vi "Read analyze results.vi"(5 "ChemStation rawdata folder":path=path "C:/Users/Optix/Dropbox (MIT)/Research/Backup/66-225 Optix data/Yiming MO/AC electrolysis/HPLC data backup", 7 "ChemStation folder":path=path "C:/Users/Optix/Dropbox (MIT)/Research/Backup/66-225 Optix data/Yiming MO/AC electrolysis/HPLC data backup", 8 "Index":dbl, 9 "Sample name":string, 10 "Experiment name":string, 11 "Exp. file path":path) -> ()   [LabVIEW 2017]
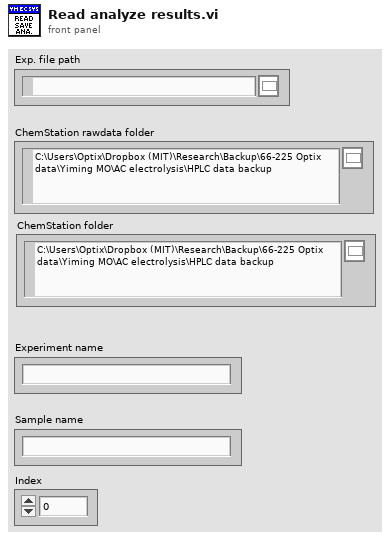
[diagram p1: front panel]
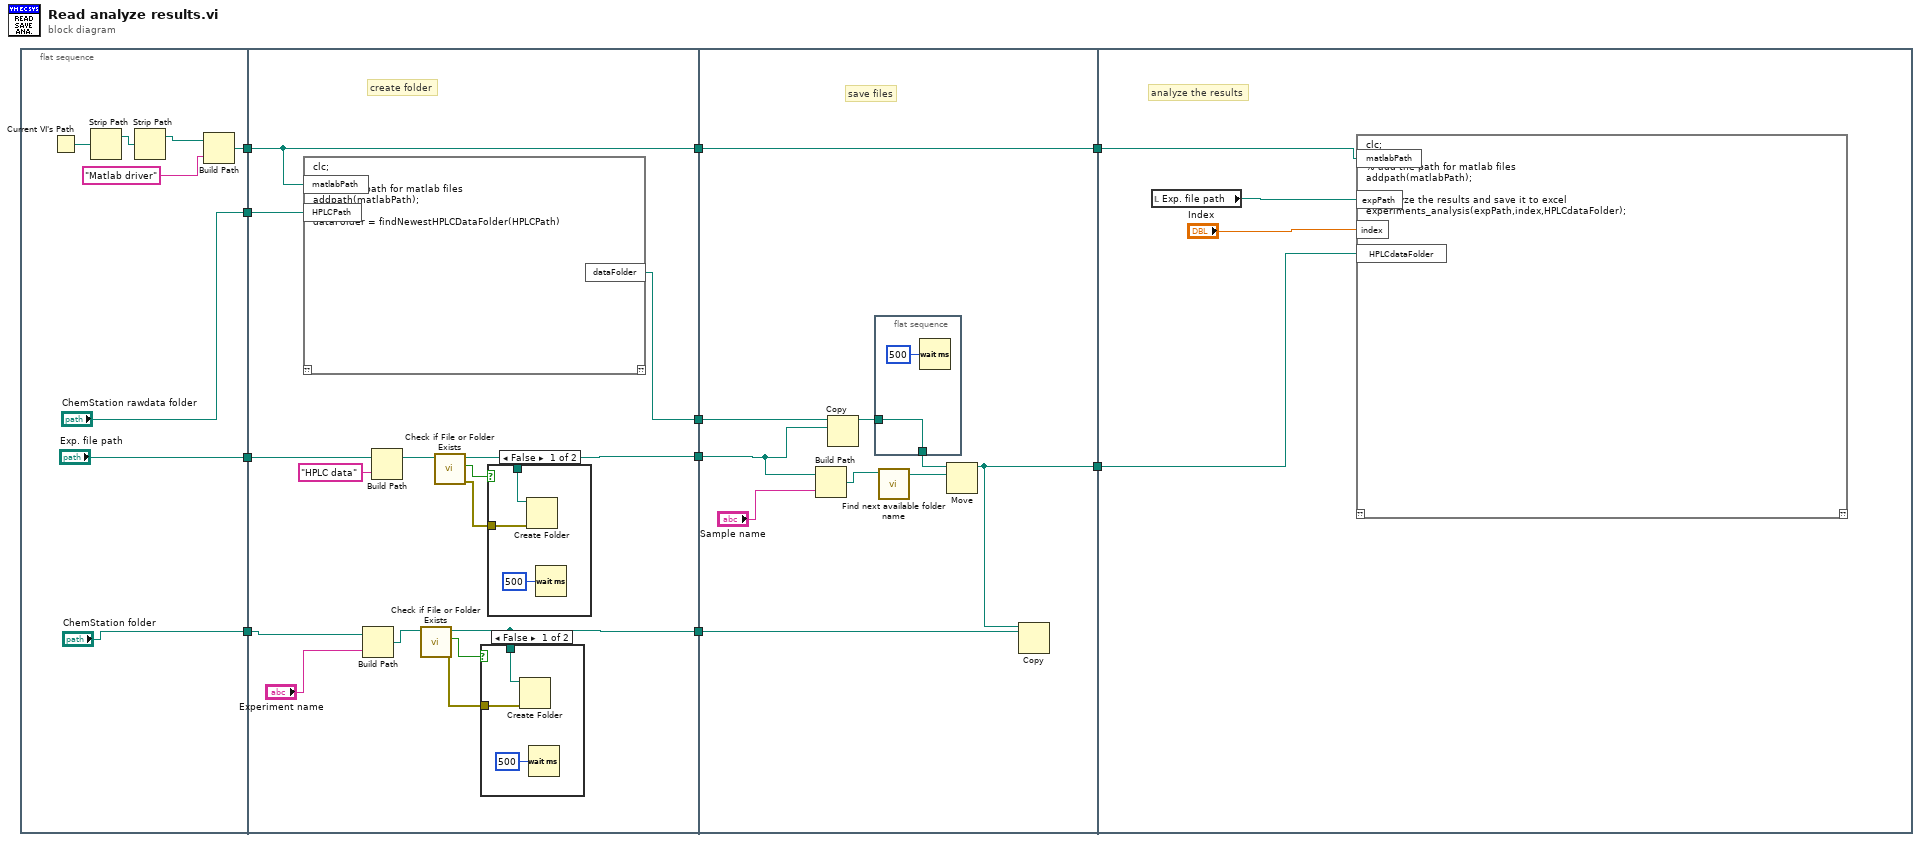
[diagram p0: block diagram]
diagram:
  n1 = flat-sequence {
    tunnel: ["Exp. file path"] -> w10
    tunnel: ["ChemStation folder"] -> w7
    tunnel: [w12] -> w3
    tunnel: ["ChemStation rawdata folder"] -> w2
    tunnel: w10 -> [w32]
    tunnel: [w29] -> w9
    tunnel: [w24] -> w8
    tunnel: w7 -> [w27]
    tunnel: [w21] -> w4
    tunnel: w3 -> [w21]
    tunnel: w2 -> [w20]
    tunnel: [w19] -> w1
    tunnel: w9 -> [w47]
    tunnel: w8 -> [w44]
    tunnel: [w41] -> w6
    tunnel: [w40] -> w5
    tunnel: w4 -> [w40]
    tunnel: w1 -> [w39]
    tunnel: w6 -> [w54]
    tunnel: w5 -> [w51]
    frame #0 {
      n2 = Current VI's Path() -> (path=w14:path)
      n3 = Strip Path(path=w14) -> (stripped path=w15:path)  [unwired: 1 out]
      n4 = Strip Path(path=w15) -> (stripped path=w16:path)  [unwired: 1 out]
      n5 = Build Path(base path=w16, name or relative path="Matlab driver") -> (appended path=w12:path)
    }
    frame #1 {
      # "create folder"
      n6 = script code="clc;\n\n% add the path for matlab files\naddpath(matlabPath);\n\ndataFolder = findNewestHPLCDataFolder(HPLCPath)"("matlabPath"=w21, "HPLCPath"=w20) -> ("dataFolder"=w19:path)  [unwired: 1 in, 1 out]
      n7 = Build Path(base path=w27, name or relative path="Experiment name") -> (appended path=w26:path)
      n8 = Build Path(base path=w32, name or relative path="HPLC data") -> (appended path=w29:path)
      n9 = call <vilib>:"Check if File or Folder Exists.vi"("path"=w26) -> ("error out"=w22:errorcluster, "file or folder exists?"=w25:bool, "dup path"=w24:path)  [unwired: 8 in]
      n10 = call <vilib>:"Check if File or Folder Exists.vi"("path"=w29) -> ("error out"=w23:errorcluster, "file or folder exists?"=w30:bool)  [unwired: 8 in, 1 out]
      n11 = case shown="False" w25 {
        tunnel: w24 -> [w35 _]
        tunnel: w22 -> [w33 _]
        frame False {
          n12 = Create Folder(path (use dialog)=w35, error in=w33) -> ()  [unwired: 1 in, 3 out]
          n13 = Wait (ms)(milliseconds to wait=u32 500) -> ()  [unwired: 1 out]
        }
        frame True {
        }
      }
      n14 = case shown="False" w30 {
        tunnel: w29 -> [w38 _]
        tunnel: w23 -> [w36 _]
        frame False {
          n15 = Create Folder(path (use dialog)=w38, error in=w36) -> ()  [unwired: 1 in, 3 out]
          n16 = Wait (ms)(milliseconds to wait=u32 500) -> ()  [unwired: 1 out]
        }
        frame True {
        }
      }
    }
    frame #2 {
      # "save files"
      n17 = Build Path(base path=w47, name or relative path="Sample name") -> (appended path=w46:path)
      n18 = Copy(10:w47, 11:w39) -> (3:w42:path)  [unwired: 3 in, 2 out]
      n19 = flat-sequence {
        tunnel: [w49] -> w43
        tunnel: w42 -> [w49]
        frame #0 {
          n20 = Wait (ms)(milliseconds to wait=u32 500) -> ()  [unwired: 1 out]
        }
      }
      n21 = call "Find next available folder name.vi"("Input folder"=w46) -> ("Output folder"=w45:path)  [unwired: 10 in]
      n22 = Move(source path=w43, 10:w45) -> (3:w41:path)  [unwired: 3 in, 2 out]
      n23 = Copy(10:w44, 11:w41) -> ()  [unwired: 3 in, 3 out]
    }
    frame #3 {
      # "analyze the results"
      n24 = local read "Exp. file path"() -> (w53:path)
      n25 = script code="clc;\n\n% add the path for matlab files\naddpath(matlabPath);\n\n% analyze the results and save it to excel\nexperiments_analysis(expPath,index,HPLCdataFolder);"("matlabPath"=w51, "expPath"=w53, "index"="Index", "HPLCdataFolder"=w54) -> ()  [unwired: 1 in, 1 out]
    }
  }
